vi "DataToArray.vi"(8 "sortie d'erreur":errorcluster, 11 "Return value":string) -> (0 "sortie d'erreur":errorcluster, 1 "String 3DArray":cluster{"Tableau":string[][]}[](array[cluster]), 2 "String 2DArray":string[][](array[string]), 3 "String 1DArray":string[](array[string]))   [LabVIEW 2020]
uses:
  <vilib>/Utility/error.llb/Error Cluster From Error Code.vi
  <vilib>/ErrorRing/Error Ring.xnode
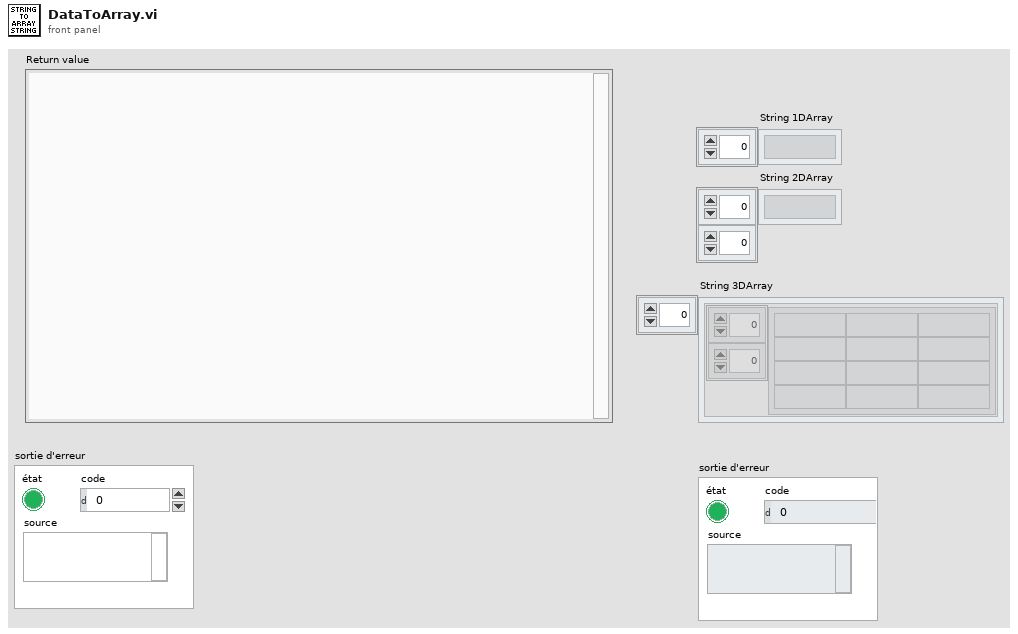
[diagram p1: front panel]
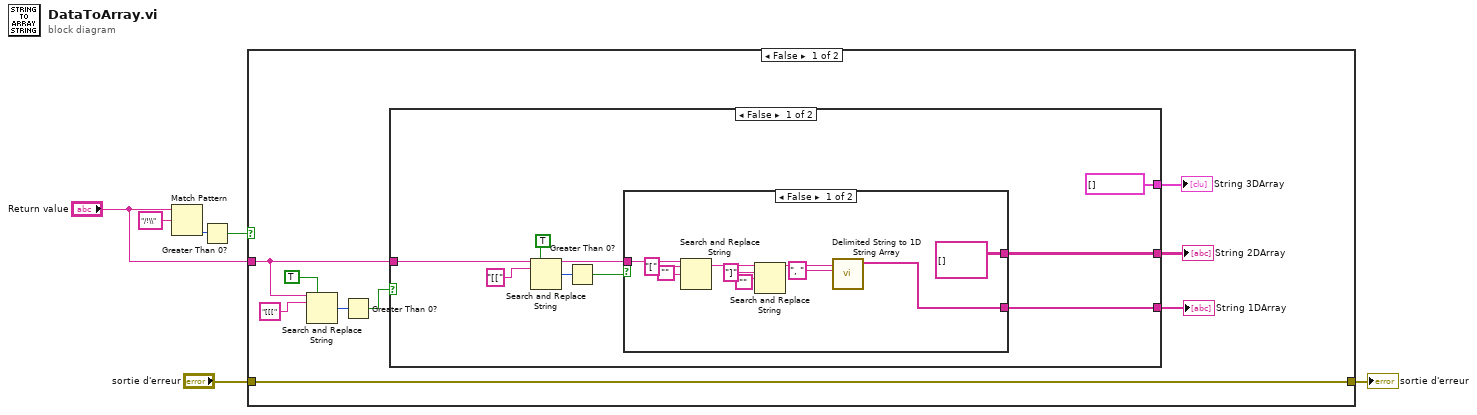
[diagram p0: block diagram]
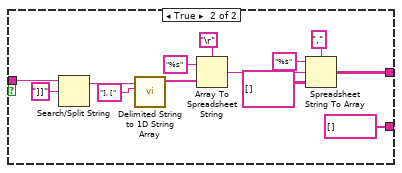
[diagram p2: hidden frame]
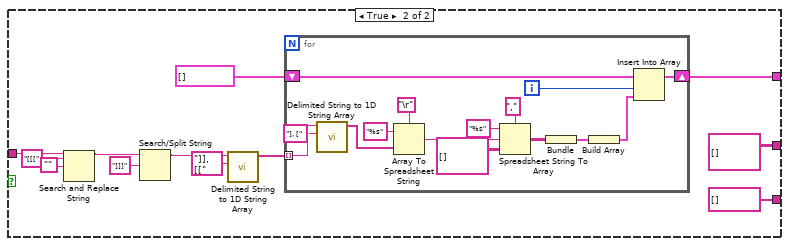
[diagram p3: hidden frame]
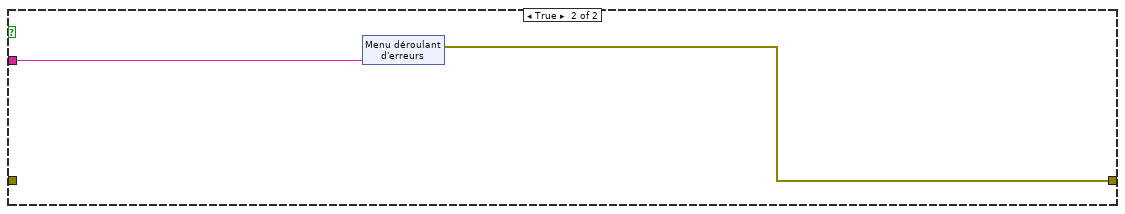
[diagram p4: hidden frame]
diagram:
  n1 = Match Pattern(string="Return value", regular expression="/!\\" ("expression régulière")) -> (offset past match=w5:i32)  [unwired: 1 in, 3 out]
  n2 = Greater Than 0?(x=w5) -> (x > 0?=w4:bool)
  n3 = case shown="False" w4 {
    tunnel: "Return value" -> [w8 w76]
    tunnel: [w7 w75] -> w3
    tunnel: "sortie d'erreur" -> [w7 _]
    frame False {
      n4 = Search and Replace String(replace all?=TRUE ("replace all? (F)"), input string=w8, search string="[[[") -> (number of replacements=w14:i32)  [unwired: 5 in, 3 out]
      n5 = Greater Than 0?(x=w14) -> (x > 0?=w13:bool)
      n6 = case shown="False" w13 {
        tunnel: w8 -> [w19 w49]
        tunnel: [w18 string[][] []] -> w10
        tunnel: [w17 string[] [] ("string array")] -> w11
        tunnel: [cluster{string[][]}[] [] w52] -> w9
        frame False {
          n7 = Search and Replace String(replace all?=TRUE ("replace all? (F)"), input string=w19, search string="[[") -> (result string=w20:string, number of replacements=w22:i32)  [unwired: 5 in, 2 out]
          n8 = Greater Than 0?(x=w22) -> (x > 0?=w21:bool)
          n9 = case shown="False" w21 {
            tunnel: w20 -> [w28 w44]
            tunnel: [string[][] [] w36] -> w18
            tunnel: [w26 string[] [] ("string array")] -> w17
            frame False {
              n10 = Search and Replace String(input string=w28, search string="[", replace string="") -> (result string=w29:string)  [unwired: 5 in, 3 out]
              n11 = Search and Replace String(input string=w29, search string="]", replace string="") -> (result string=w27:string)  [unwired: 5 in, 3 out]
              n12 = call <vilib>:"Delimited String to 1D String Array.vi"("delimiter"=", ", "delimited string"=w27) -> ("string array"=w26:string[])  [unwired: 9 in]
            }
            frame True {
              n13 = Search/Split String(string=w44, search string/char (-)="]]" ("chaîne/car. recherché (-)")) -> (substring before match=w43:string)  [unwired: 1 in, 2 out]
              n14 = call <vilib>:"Delimited String to 1D String Array.vi"("delimiter"="], [", "delimited string"=w43) -> ("string array"=w46:string[])  [unwired: 9 in]
              n15 = Array To Spreadsheet String(delimiter (Tab)="\r", array=w46, 3:"%s" ("chaîne de format")) -> (spreadsheet string=w37:string)
              n16 = Spreadsheet String To Array(delimiter (Tab)="," ("séparateur (Tabulation)"), format string="%s" ("chaîne de format"), spreadsheet string=w37, array type (2D Dbl)=string[][] []) -> (array=w36:string[][])
            }
          }
        }
        frame True {
          n17 = Search and Replace String(input string=w49, search string="[[[", replace string="") -> (result string=w48:string)  [unwired: 5 in, 3 out]
          n18 = Search/Split String(string=w48, search string/char (-)="]]]" ("chaîne/car. recherché (-)")) -> (substring before match=w53:string)  [unwired: 1 in, 2 out]
          n19 = call <vilib>:"Delimited String to 1D String Array.vi"("delimiter"="]], [[", "delimited string"=w53) -> ("string array"=w56:string[])  [unwired: 9 in]
          n20 = for {
            tunnel: w56 -> [w71] mode=indexing
            shift-right: [w60] -> w52
            shift-left: cluster{string[][]}[] [] -> [w61]
            i -> [w62]
            n21 = call <vilib>:"Delimited String to 1D String Array.vi"("delimiter"="], [", "delimited string"=w71) -> ("string array"=w67:string[])  [unwired: 9 in]
            n22 = Array To Spreadsheet String(delimiter (Tab)="\r", array=w67, 3:"%s" ("chaîne de format")) -> (spreadsheet string=w66:string)
            n23 = Spreadsheet String To Array(delimiter (Tab)="," ("séparateur (Tabulation)"), format string="%s" ("chaîne de format"), spreadsheet string=w66, array type (2D Dbl)=string[][] []) -> (array=w65:string[][])
            n24 = Bundle(w65) -> (w64:cluster{string[][]})  [unwired: 1 in]
            n25 = Build Array(w64) -> (w63:cluster{string[][]}[])
            n26 = Insert Into Array(array=w61, index=w62, new element=w63) -> (w60:cluster{string[][]}[])
          }
        }
      }
      "String 1DArray" <- w11
      "String 2DArray" <- w10
      "String 3DArray" <- w9
    }
    frame True {
      n27 = xnode "Menu déroulant d'erreurs"("parameter 0"=w76) -> ("error out"=w75:errorcluster)
    }
  }
  "sortie d'erreur" <- w3
